vi "rdb_json_decode.vi"(8 "error in (no error)":errorcluster, 11 "json":string) -> (0 "error out":errorcluster, 3 "elements":T1[](array[typedef]))   [LabVIEW 2017]
uses:
  rdb_json_element.ctl
  rdb_json_type.ctl
  <vilib>/regexp/Match Regular Expression.xnode
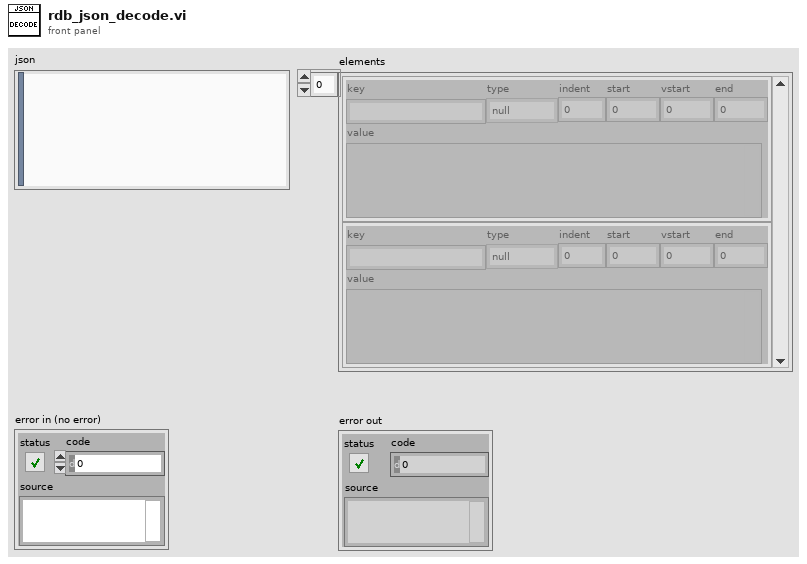
[diagram p1: front panel]
types:
  T1 = typedef "rdb_json_element.ctl" = cluster{"key":string, "type":T2, "indent":i32, "start":i32, "vstart":i32, "end":i32, "value":variant}
  T2 = typedef "rdb_json_type.ctl" = enum8{"null", "bool", "int", "uint", "float", "string", "array", "object", "invalid"}
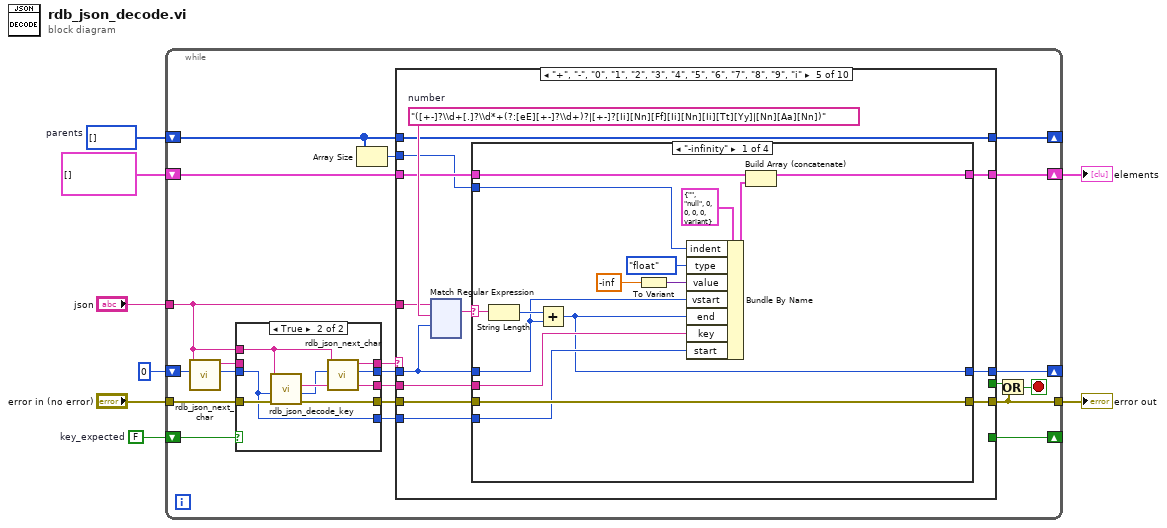
[diagram p0: block diagram]
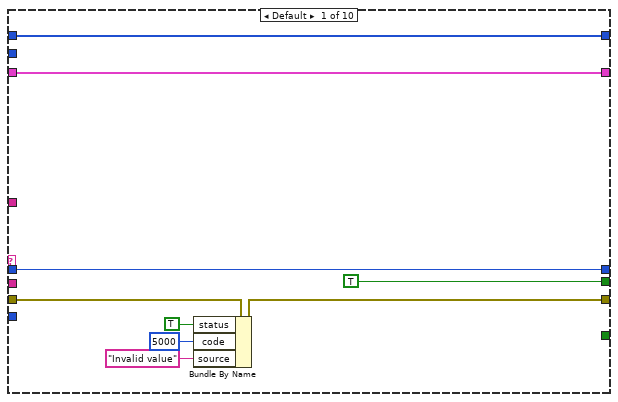
[diagram p2: hidden frame]
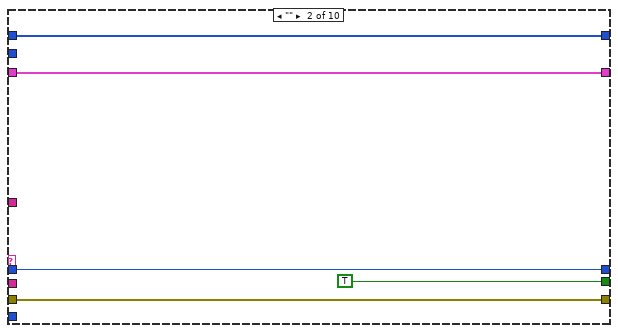
[diagram p3: hidden frame]
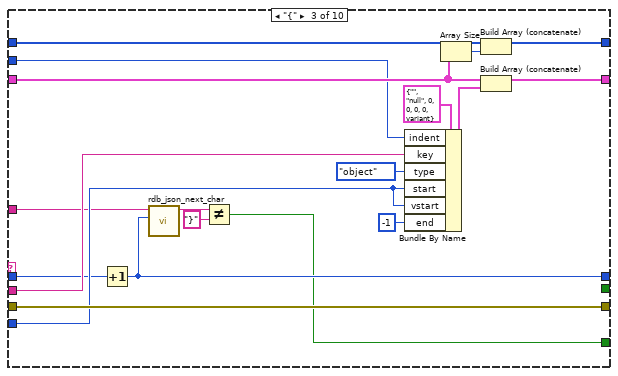
[diagram p4: hidden frame]
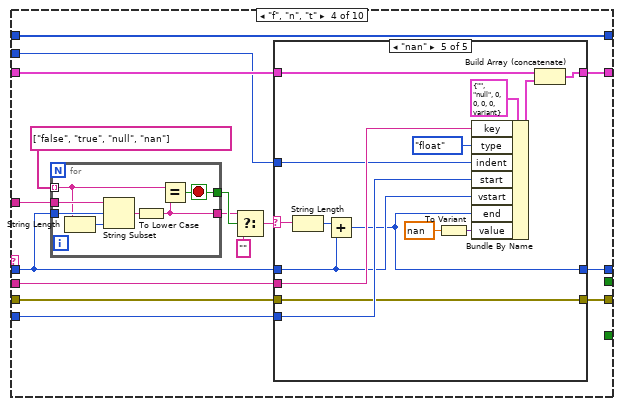
[diagram p5: hidden frame]
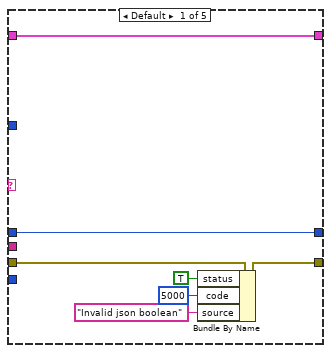
[diagram p6: hidden frame]
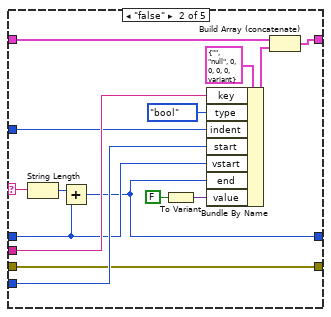
[diagram p7: hidden frame]
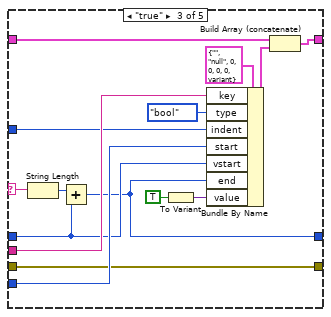
[diagram p8: hidden frame]
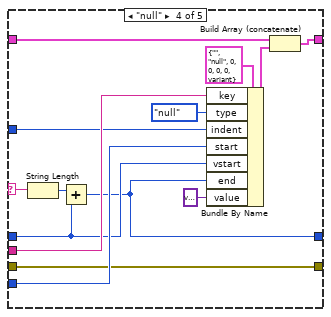
[diagram p9: hidden frame]
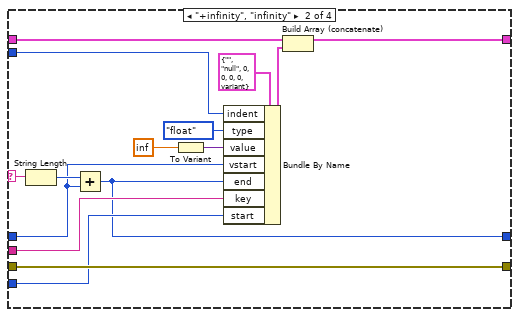
[diagram p10: hidden frame]
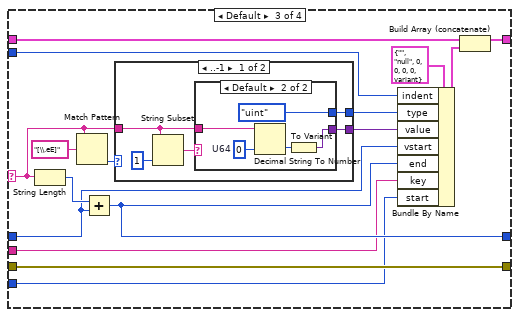
[diagram p11: hidden frame]
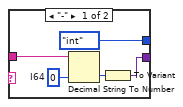
[diagram p12: hidden frame]
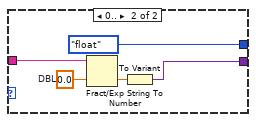
[diagram p13: hidden frame]
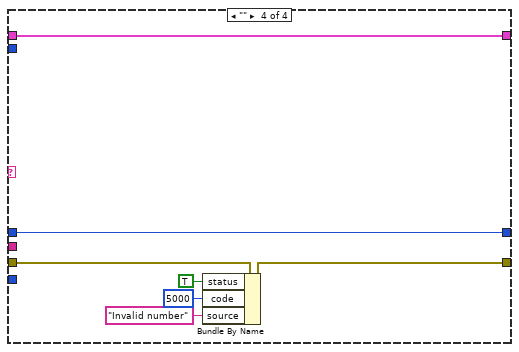
[diagram p14: hidden frame]
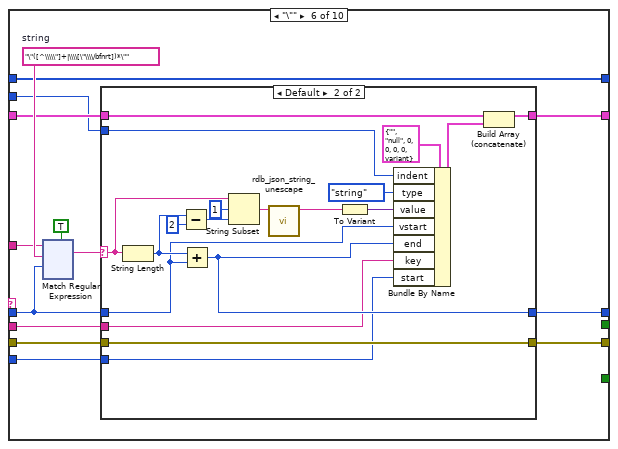
[diagram p15: hidden frame]
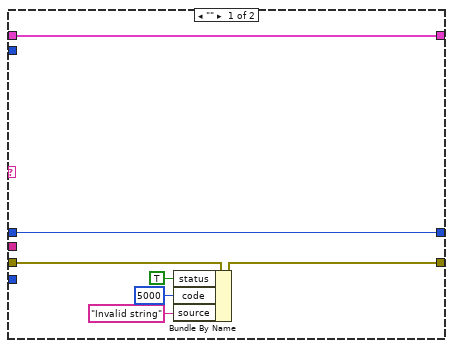
[diagram p16: hidden frame]
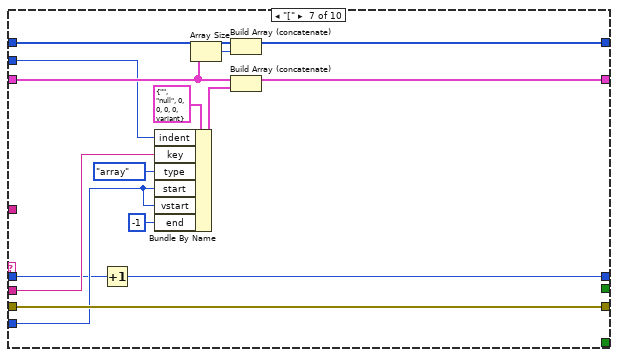
[diagram p17: hidden frame]
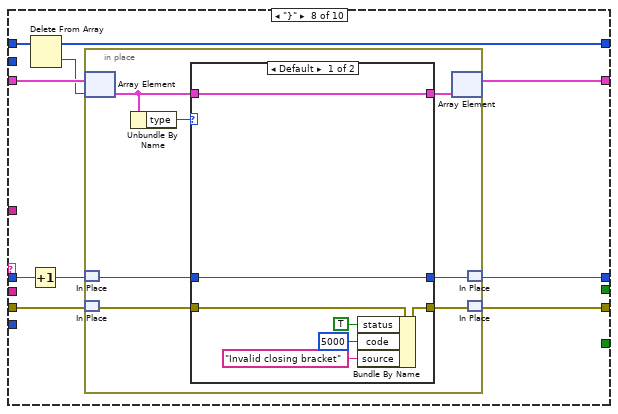
[diagram p18: hidden frame]
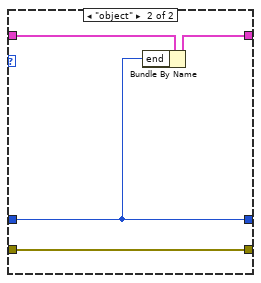
[diagram p19: hidden frame]
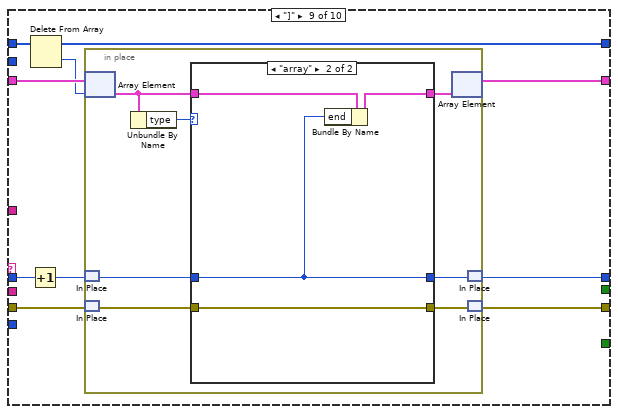
[diagram p20: hidden frame]
diagram:
  w2 = i32[] []  # parents
  w1 = FALSE  # key_expected
  n1 = while {
    tunnel: "json" -> [w13]
    shift-right: [w15] -> _
    shift-left: 0 ("offset (0)") -> [w29]
    shift-right: [w14] -> _
    shift-left: w1 -> [w26]
    tunnel: "error in (no error)" -> [w28]
    shift-right: [w18] -> w5
    shift-left: T1[] [] ("elements") -> [w21]
    tunnel: [w12] -> w3
    shift-right: [w20] -> _
    shift-left: w2 -> [w19]
    stop <- w10 stop-if-true
    n2 = call "rdb_json_next_char.vi"("offset (0)"=w29, "json"=w13) -> ("offset before char"=w27:i32, "non-whitespace char"=w25:string)  [unwired: 8 in]
    n3 = case shown="True" w26 {
      tunnel: w28 -> [w599 w607]
      tunnel: w13 -> [_ w601]
      tunnel: w27 -> [w597 w600]
      tunnel: [w599 w606] -> w24
      tunnel: [_ w605] -> w17
      tunnel: w25 -> [w598 _]
      tunnel: [w597 w603] -> w22
      tunnel: [w598 w602] -> w23
      tunnel: [w597 w600] -> w16
      frame False {
      }
      frame True {
        n4 = call "rdb_json_decode_key.vi"("error in (no error)"=w607, "offset (0)"=w600, "data"=w601) -> ("error out"=w606:errorcluster, "offset past match"=w604:i32, "key"=w605:string)  [unwired: 6 in]
        n5 = call "rdb_json_next_char.vi"("offset (0)"=w604, "json"=w601) -> ("offset before char"=w603:i32, "non-whitespace char"=w602:string)  [unwired: 8 in]
      }
    }
    n6 = Array Size(array=w19) -> (size(s)=w9:i32)
    n7 = case shown="\"+\", \"-\", \"0\", \"1\", \"2\", \"3\", \"4\", \"5\", \"6\", \"7\", \"8\", \"9\", \"i\"" w23 {
      tunnel: w24 -> [w35 w39 w62 w73 w162 w362 w520 w522 w550 w596]
      tunnel: w22 -> [w33 w43 w50 w70 w160 w360 w509 w527 w555 w595]
      tunnel: [w34 w39 w62 w74 w157 w361 w520 w521 w549 w596] -> w12
      tunnel: w21 -> [w31 w41 w59 w78 w158 w357 w517 w529 w557 w592]
      tunnel: [w32 w42 w61 w64 w153 w353 w519 w530 w558 w594] -> w20
      tunnel: w19 -> [w32 w42 w45 w64 w153 w353 w507 w526 w554 w594]
      tunnel: [w31 w41 w58 w77 w159 w358 w516 w528 w556 w592] -> w18
      tunnel: w17 -> [_ _ w56 w76 w155 w355 w514 _ _ _]
      tunnel: w16 -> [_ _ w53 w75 w154 w354 w511 _ _ _]
      tunnel: [w33 w43 w49 w72 w156 w356 w508 w523 w551 w578] -> w15
      tunnel: [_ _ w46 _ _ _ _ _ _ w579] -> w14
      tunnel: w13 -> [_ _ w51 w71 w161 w359 _ _ _ w587]
      tunnel: [TRUE TRUE _ _ _ _ _ _ _ _] -> w11
      tunnel: w9 -> [_ _ w44 w63 w152 w352 w506 _ _ w577]
      frame Default {
        n8 = Bundle By Name(cluster=w35, "status"=TRUE, "code"=5000, "source"="Invalid value") -> (w34:errorcluster)
      }
      frame "" {
      }
      frame "{" {
        n9 = Increment(x=w50) -> (x+1=w49:i32)
        n10 = call "rdb_json_next_char.vi"("offset (0)"=w49, "json"=w51) -> ("non-whitespace char"=w48:string)  [unwired: 8 in, 1 out]
        n11 = Not Equal?(x=w48, y="}") -> (x != y?=w46:bool)
        n12 = Bundle By Name(cluster=T1 {"key"="", "type"=enum."null", "indent"=0, "start"=0, "vstart"=0, "end"=0, "value"=variant} ("element"), "indent"=w44, "key"=w56, "type"=rdb_json_type."object", "start"=w53, "vstart"=w53, "end"=-1) -> (w54:T1)
        n13 = Array Size(array=w59) -> (size(s)=w60:i32)
        n14 = Build Array (concatenate)(w45, w60) -> (w61:i32[])
        n15 = Build Array (concatenate)(w59, w54) -> (w58:T1[])
      }
      frame "f", "n", "t" {
        n16 = for {
          tunnel: w71 -> [w85]
          tunnel: w70 -> [w83]
          tunnel: string[] ["false", "true", "null", "nan"] -> [w82] mode=indexing
          tunnel: [w80] -> w67
          tunnel: [w79] -> w68
          stop <- w79 stop-if-true
          n17 = String Length(string=w82) -> (length=w84:i32)
          n18 = String Subset(string=w85, offset (0)=w83, length (rest)=w84) -> (substring=w81:string)
          n19 = To Lower Case(string=w81) -> (all lower case string=w80:string)
          n20 = Equal?(x=w82, y=w80) -> (x = y?=w79:bool)
        }
        n21 = Select(t=w67, s=w68, f="") -> (s? t:f=w65:string)
        n22 = case shown="\"nan\"" w65 {
          selector: w65 -> [_ w96 w111 w127 w142]
          tunnel: w78 -> [w92 w107 w122 w136 w151]
          tunnel: [w92 w106 w121 w135 w150] -> w77
          tunnel: w76 -> [_ w104 w119 w133 w148]
          tunnel: w63 -> [_ w101 w116 w130 w145]
          tunnel: w75 -> [_ w100 w115 w129 w144]
          tunnel: w70 -> [w86 w94 w109 w125 w140]
          tunnel: [w90 w99 w114 w128 w143] -> w74
          tunnel: w73 -> [w91 w99 w114 w128 w143]
          tunnel: [w86 w93 w108 w124 w139] -> w72
          frame Default {
            n23 = Bundle By Name(cluster=w91, "status"=TRUE, "code"=5000, "source"="Invalid json boolean") -> (w90:errorcluster)
          }
          frame "false" {
            n24 = String Length(string=w96) -> (length=w95:i32)
            n25 = Add(x=w95, y=w94) -> (x+y=w93:i32)
            n26 = To Variant(anything=FALSE) -> (Variant=w97:variant)
            n27 = Bundle By Name(cluster=T1 {"key"="", "type"=enum."null", "indent"=0, "start"=0, "vstart"=0, "end"=0, "value"=variant} ("element"), "key"=w104, "type"=rdb_json_type."bool", "indent"=w101, "start"=w100, "vstart"=w94, "end"=w93, "value"=w97) -> (w103:T1)
            n28 = Build Array (concatenate)(w107, w103) -> (w106:T1[])
          }
          frame "true" {
            n29 = String Length(string=w111) -> (length=w110:i32)
            n30 = Add(x=w110, y=w109) -> (x+y=w108:i32)
            n31 = To Variant(anything=TRUE) -> (Variant=w112:variant)
            n32 = Bundle By Name(cluster=T1 {"key"="", "type"=enum."null", "indent"=0, "start"=0, "vstart"=0, "end"=0, "value"=variant} ("element"), "key"=w119, "type"=rdb_json_type."bool", "indent"=w116, "start"=w115, "vstart"=w109, "end"=w108, "value"=w112) -> (w118:T1)
            n33 = Build Array (concatenate)(w122, w118) -> (w121:T1[])
          }
          frame "null" {
            n34 = String Length(string=w127) -> (length=w126:i32)
            n35 = Add(x=w126, y=w125) -> (x+y=w124:i32)
            n36 = Bundle By Name(cluster=T1 {"key"="", "type"=enum."null", "indent"=0, "start"=0, "vstart"=0, "end"=0, "value"=variant} ("element"), "key"=w133, "type"=rdb_json_type."null", "indent"=w130, "start"=w129, "vstart"=w125, "end"=w124, "value"=variant) -> (w132:T1)
            n37 = Build Array (concatenate)(w136, w132) -> (w135:T1[])
          }
          frame "nan" {
            n38 = String Length(string=w142) -> (length=w141:i32)
            n39 = Add(x=w141, y=w140) -> (x+y=w139:i32)
            n40 = To Variant(anything=nan) -> (Variant=w137:variant)
            n41 = Bundle By Name(cluster=T1 {"key"="", "type"=enum."null", "indent"=0, "start"=0, "vstart"=0, "end"=0, "value"=variant} ("element"), "key"=w148, "type"=rdb_json_type."float", "indent"=w145, "start"=w144, "vstart"=w140, "end"=w139, "value"=w137) -> (w147:T1)
            n42 = Build Array (concatenate)(w151, w147) -> (w150:T1[])
          }
        }
      }
      frame "+", "-", "0", "1", "2", "3", "4", "5", "6", "7", "8", "9", "i" {
        w164 = "([+-]?\\d+[.]?\\d*+(?:[eE][+-]?\\d+)?|[+-]?[Ii][Nn][Ff][Ii][Nn][Ii][Tt][Yy]|[Nn][Aa][Nn])"  # number
        n43 = xnode "Match Regular Expression"("input string"=w161, "regular expression"=w164, "offset (0)"=w160) -> ("whole match"=w163:string)  [unwired: 3 in, 4 out]
        n44 = case shown="\"-infinity\"" w163 {
          selector: w163 -> [w177 w192 w200 _]
          tunnel: [w178 w193 w209 w233] -> w157
          tunnel: w162 -> [w178 w193 w209 w234]
          tunnel: w160 -> [w167 w182 w198 w232]
          tunnel: [w166 w181 w197 w232] -> w156
          tunnel: [w174 w189 w205 w231] -> w159
          tunnel: w158 -> [w175 w190 w206 w231]
          tunnel: w152 -> [w169 w184 w201 _]
          tunnel: w155 -> [w171 w186 w196 _]
          tunnel: w154 -> [w168 w183 w195 _]
          frame "-infinity" {
            n45 = String Length(string=w177) -> (length=w176:i32)
            n46 = Add(x=w176, y=w167) -> (x+y=w166:i32)
            n47 = To Variant(anything=-inf) -> (Variant=w165:variant)
            n48 = Bundle By Name(cluster=T1 {"key"="", "type"=enum."null", "indent"=0, "start"=0, "vstart"=0, "end"=0, "value"=variant} ("element"), "indent"=w169, "type"=rdb_json_type."float", "value"=w165, "vstart"=w167, "end"=w166, "key"=w171, "start"=w168) -> (w172:T1)
            n49 = Build Array (concatenate)(w175, w172) -> (w174:T1[])
          }
          frame "+infinity", "infinity" {
            n50 = String Length(string=w192) -> (length=w191:i32)
            n51 = Add(x=w191, y=w182) -> (x+y=w181:i32)
            n52 = To Variant(anything=inf) -> (Variant=w180:variant)
            n53 = Bundle By Name(cluster=T1 {"key"="", "type"=enum."null", "indent"=0, "start"=0, "vstart"=0, "end"=0, "value"=variant} ("element"), "indent"=w184, "type"=rdb_json_type."float", "value"=w180, "vstart"=w182, "end"=w181, "key"=w186, "start"=w183) -> (w187:T1)
            n54 = Build Array (concatenate)(w190, w187) -> (w189:T1[])
          }
          frame Default {
            n55 = String Length(string=w200) -> (length=w199:i32)
            n56 = Match Pattern(string=w200, regular expression="[\\.eE]") -> (offset past match=w208:i32)  [unwired: 1 in, 3 out]
            n57 = Add(x=w199, y=w198) -> (x+y=w197:i32)
            n58 = case shown="..-1" w208 {
              tunnel: w200 -> [w214 w230]
              tunnel: [w213 w227] -> w202
              tunnel: [w211 rdb_json_type."float" ("type")] -> w203
              frame ..-1 {
                n59 = String Subset(string=w214, length (rest)=1 ("length (rest)")) -> (substring=w212:string)  [unwired: 1 in]
                n60 = case shown="Default" w212 {
                  tunnel: w214 -> [w220 w225]
                  tunnel: [w217 w222] -> w213
                  tunnel: [rdb_json_type."int" ("type") rdb_json_type."uint" ("type")] -> w211
                  frame "-" {
                    w219 = i64 0  # I64
                    n61 = Decimal String To Number(string=w220, default (0L)=w219) -> (number=w218:i64)  [unwired: 1 in, 1 out]
                    n62 = To Variant(anything=w218) -> (Variant=w217:variant)
                  }
                  frame Default {
                    w224 = u64 0  # U64
                    n63 = Decimal String To Number(string=w225, default (0L)=w224) -> (number=w223:u64)  [unwired: 1 in, 1 out]
                    n64 = To Variant(anything=w223) -> (Variant=w222:variant)
                  }
                }
              }
              frame 0.. {
                w229 = 0.0  # DBL
                n65 = Fract/Exp String To Number(string=w230, default (0 dbl)=w229) -> (number=w228:dbl)  [unwired: 2 in, 1 out]
                n66 = To Variant(anything=w228) -> (Variant=w227:variant)
              }
            }
            n67 = Bundle By Name(cluster=T1 {"key"="", "type"=enum."null", "indent"=0, "start"=0, "vstart"=0, "end"=0, "value"=variant} ("element"), "indent"=w201, "type"=w203, "value"=w202, "vstart"=w198, "end"=w197, "key"=w196, "start"=w195) -> (w204:T1)
            n68 = Build Array (concatenate)(w206, w204) -> (w205:T1[])
          }
          frame "" {
            n69 = Bundle By Name(cluster=w234, "status"=TRUE, "code"=5000, "source"="Invalid number") -> (w233:errorcluster)
          }
        }
      }
      frame "\"" {
        w365 = "\"([^\\\\\"]+|\\\\[\"\\\\/bfnrt])*\""  # string
        n70 = xnode ("Match Regular Expression")("input string"=w359, "regular expression"=w365, "offset (0)"=w360, "multiline? (F)"=TRUE) -> ("whole match"=w363:string)  [unwired: 2 in, 4 out]
        n71 = case shown="Default" w363 {
          selector: w363 -> [_ w386]
          tunnel: [w371 w387] -> w361
          tunnel: w362 -> [w372 w387]
          tunnel: w360 -> [w367 w377]
          tunnel: [w367 w376] -> w356
          tunnel: [w366 w383] -> w358
          tunnel: w357 -> [w366 w384]
          tunnel: w352 -> [_ w381]
          tunnel: w355 -> [_ w375]
          tunnel: w354 -> [_ w374]
          frame "" {
            n72 = Bundle By Name(cluster=w372, "status"=TRUE, "code"=5000, "source"="Invalid string") -> (w371:errorcluster)
          }
          frame Default {
            n73 = String Length(string=w386) -> (length=w385:i32)
            n74 = Subtract(x=w385, y=2) -> (x-y=w388:i32)
            n75 = Add(x=w385, y=w377) -> (x+y=w376:i32)
            n76 = String Subset(string=w386, offset (0)=1, length (rest)=w388) -> (substring=w391:string)
            n77 = call "rdb_json_string_unescape.vi"("escaped string"=w391) -> ("string out"=w379:string)  [unwired: 9 in, 1 out]
            n78 = To Variant(anything=w379) -> (Variant=w378:variant)
            n79 = Bundle By Name(cluster=T1 {"key"="", "type"=enum."null", "indent"=0, "start"=0, "vstart"=0, "end"=0, "value"=variant} ("element"), "indent"=w381, "type"=rdb_json_type."string", "value"=w378, "vstart"=w377, "end"=w376, "key"=w375, "start"=w374) -> (w373:T1)
            n80 = Build Array (concatenate)(w384, w373) -> (w383:T1[])
          }
        }
      }
      frame "[" {
        n81 = Increment(x=w509) -> (x+1=w508:i32)
        n82 = Bundle By Name(cluster=T1 {"key"="", "type"=enum."null", "indent"=0, "start"=0, "vstart"=0, "end"=0, "value"=variant} ("element"), "indent"=w506, "key"=w514, "type"=rdb_json_type."array", "start"=w511, "vstart"=w511, "end"=-1) -> (w512:T1)
        n83 = Array Size(array=w517) -> (size(s)=w518:i32)
        n84 = Build Array (concatenate)(w507, w518) -> (w519:i32[])
        n85 = Build Array (concatenate)(w517, w512) -> (w516:T1[])
      }
      frame "}" {
        n86 = Increment(x=w527) -> (x+1=w524:i32)
        n87 = Delete From Array(array=w526) -> (deleted portion=w525:i32, array with subset deleted=w530:i32[])  [unwired: 2 in]
        n88 = in-place {
          n89 = in-place-array #1(w529, w525) -> (w536:T1)
          n90 = in-place-match #2(w524) -> (w535:i32)
          n91 = in-place-match #3(w522) -> (w533:errorcluster)
          n92 = Unbundle By Name(w536) -> ("type"=w531:T2)
          n93 = case shown="Default" w531 {
            tunnel: [w538 w548] -> w537
            tunnel: w536 -> [w538 w547]
            tunnel: w535 -> [w544 w545]
            tunnel: [w542 w546] -> w534
            tunnel: w533 -> [w543 w546]
            tunnel: [w544 w545] -> w532
            frame Default {
              n94 = Bundle By Name(cluster=w543, "status"=TRUE, "code"=5000, "source"="Invalid closing bracket") -> (w542:errorcluster)
            }
            frame "object" {
              n95 = Bundle By Name(cluster=w547, "end"=w545) -> (w548:T1)
            }
          }
          n96 = in-place-array #1(w537) -> (w528:T1[])  [unwired: 1 out]
          n97 = in-place-match #2(w532) -> (w523:i32)
          n98 = in-place-match #3(w534) -> (w521:errorcluster)
        }
      }
      frame "]" {
        n99 = Increment(x=w555) -> (x+1=w552:i32)
        n100 = Delete From Array(array=w554) -> (deleted portion=w553:i32, array with subset deleted=w558:i32[])  [unwired: 2 in]
        n101 = in-place {
          n102 = in-place-array #4(w557, w553) -> (w564:T1)
          n103 = in-place-match #5(w552) -> (w563:i32)
          n104 = in-place-match #6(w550) -> (w561:errorcluster)
          n105 = Unbundle By Name(w564) -> ("type"=w559:T2)
          n106 = case shown="\"array\"" w559 {
            tunnel: [w566 w576] -> w565
            tunnel: w564 -> [w566 w575]
            tunnel: w563 -> [w572 w573]
            tunnel: [w570 w574] -> w562
            tunnel: w561 -> [w571 w574]
            tunnel: [w572 w573] -> w560
            frame Default {
              n107 = Bundle By Name(cluster=w571, "status"=TRUE, "code"=5000, "source"="Invalid closing bracket") -> (w570:errorcluster)
            }
            frame "array" {
              n108 = Bundle By Name(cluster=w575, "end"=w573) -> (w576:T1)
            }
          }
          n109 = in-place-array #4(w565) -> (w556:T1[])  [unwired: 1 out]
          n110 = in-place-match #5(w560) -> (w551:i32)
          n111 = in-place-match #6(w562) -> (w549:errorcluster)
        }
      }
      frame "," {
        n112 = Increment(x=w595) -> (x+1=w578:i32)
        n113 = Decrement(x=w577) -> (x-1=w593:i32)
        n114 = call "rdb_json_next_char.vi"("offset (0)"=w578, "json"=w587) -> ("non-whitespace char"=w584:string)  [unwired: 8 in, 1 out]
        n115 = Index Array(array=w594, index=w593) -> (element=w591:i32)
        n116 = Equal?(x=w584, y="]") -> (x = y?=w583:bool)
        n117 = Equal?(x=w584, y="}") -> (x = y?=w582:bool)
        n118 = Index Array(array=w592, index=w591) -> (element=w590:T1)
        n119 = Or(x=w583, y=w582) -> (x .or. y?=w580:bool)
        n120 = Unbundle By Name(w590) -> ("type"=w589:T2)
        n121 = Equal?(x=w589, y=rdb_json_type."object") -> (x = y?=w581:bool)
        n122 = Compound Arithmetic op=AND(w581, invert w580) -> (w579:bool)
      }
    }
    n123 = Or(x=w11, y=w12) -> (x .or. y?=w10:bool)
  }
  "error out" <- w3
  "elements" <- w5
